vi "ke37xx Close Channels.vi"(0 "VISA Resource Name":refnum<visa-resource-name>, 1 "Channel List":string, 7 "Mode (0: Normal)":enum16{"Normal", "Exclusive", "Slot Exclusive"}(ring), 11 "error in (no error)":errorcluster) -> (4 "VISA Resource Name Out":refnum<visa-resource-name>, 15 "error out":errorcluster)   [LabVIEW 2009, in "Keithley 3700 Series.lvlib"]
doc: "This VI allows you to close a specific channels. You can close channels in normal mode, exclusive mode, or slot exclusive mode."
uses:
  <instrlib>/Keithley 3706/Keithley 3700 Series.lvlib
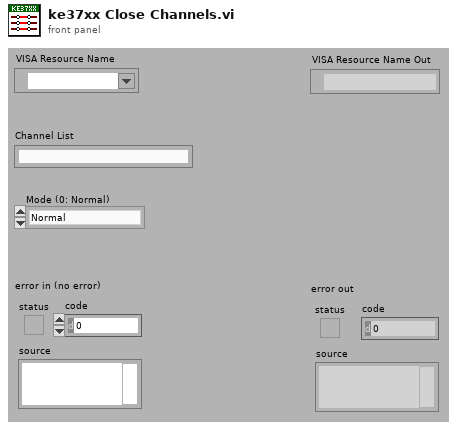
[diagram p1: front panel]
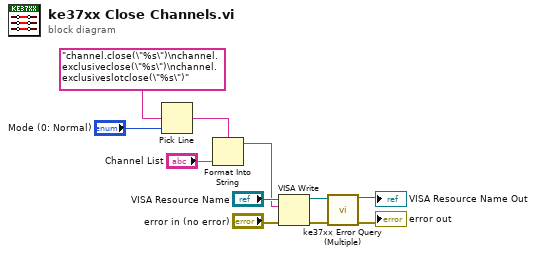
[diagram p0: block diagram]
diagram:
  n1 = Pick Line(multi-line string="channel.close(\"%s\")\nchannel.exclusiveclose(\"%s\")\nchannel.exclusiveslotclose(\"%s\")", line index="Mode (0: Normal)") -> (output string=w8:string)  [unwired: 1 out]
  n2 = Format Into String(format string=w8, "Channel List") -> (resulting string=w5:string)  [unwired: 2 in, 1 out]
  n3 = VISA Write(VISA resource name="VISA Resource Name", write buffer=w5, error in (no error)="error in (no error)") -> (VISA resource name out=w4:refnum<visa-resource-name>, error out=w2:errorcluster)  [unwired: 1 out]
  n4 = call <instrlib>:"ke37xx Error Query (Multiple).vi"("VISA resource name"=w4, "error in (no error)"=w2) -> ("VISA resource name out"=→"VISA Resource Name Out":refnum<visa-resource-name>, "error out"=→"error out":errorcluster)  [unwired: 12 out]
